vi "Update Metadata using listbox names.vi"(6 "loadStatus Refnum":refnum<vi>, 8 "error in":errorcluster, 10 "Site":string, 11 "RefNumArrIn":refnum<vi>[](array[refnum])) -> (0 "error out":errorcluster, 3 "RefNumArrOut":refnum<vi>[](array[refnum]))   [LabVIEW 2015]
uses:
  <vilib>/addons/database/Connection.llb/DB Tools Open Connec (Path).vi
  <vilib>/addons/database/Connection.llb/Conn Execute.vi
  <vilib>/addons/database/Recordset.llb/Rec Destroy - Connection.vi
  <vilib>/addons/database/NI_Database_API.lvlib
panel:
  out "App.Dir":path
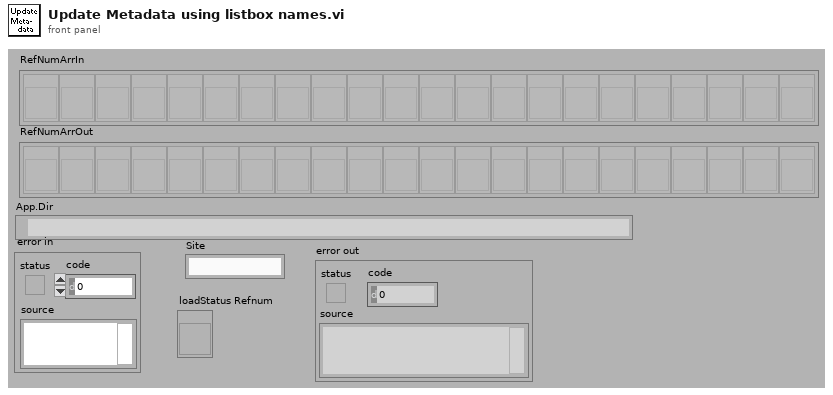
[diagram p1: front panel]
types:
  T1 = typedef "NI_Database_API.lvlib/Conn ObjectReference.ctl" = refnum<k1>
  T2 = typedef "NI_Database_API.lvlib/Rec ObjectReference.ctl" = refnum<k1>
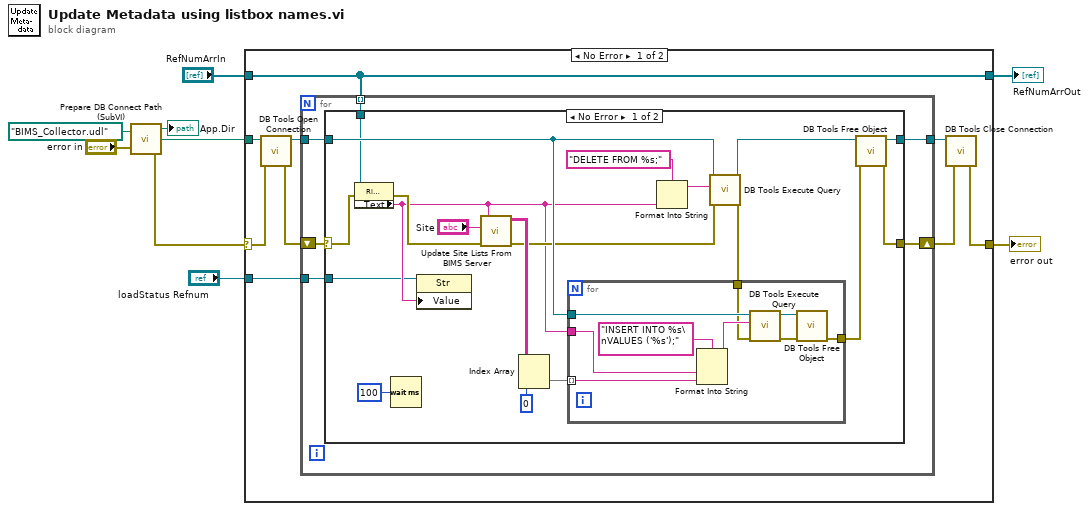
[diagram p0: block diagram]
diagram:
  n1 = call "Prepare DB Connect Path (SubVI).vi"("connectString"=path "BIMS_Collector.udl", "error in"="error in") -> ("App.Dir"=→"App.Dir":path, "appended path"=w9:path, "error out"=w3:errorcluster)
  n2 = case shown="No Error" w3 {
    selector: w3 -> [w13 w55]
    tunnel: w9 -> [w16 _]
    tunnel: [w12 w55] -> w2
    tunnel: "RefNumArrIn" -> [w11 w56]
    tunnel: [w11 w56] -> w6
    tunnel: "loadStatus Refnum" -> [w10 _]
    frame No Error {
      n3 = call-poly <vilib>:"DB Tools Open Connection.vi"("error in (no error)"=w13, "connection information"=w16) -> ("error out"=w18:errorcluster, "connection reference"=w17:T1)  [unwired: 3 in, 3 out]
      n4 = for {
        shift-right: [w23] -> w14
        shift-left: w18 -> [w21]
        tunnel: w17 -> [w22]
        tunnel: [w24] -> w15
        tunnel: w11 -> [w20] mode=indexing
        tunnel: w10 -> [w19]
        n5 = case shown="No Error" w21 {
          selector: w21 -> [w28 w53]
          tunnel: [w43 w54] -> w24
          tunnel: [w42 w53] -> w23
          tunnel: w22 -> [w40 w54]
          tunnel: w20 -> [w30 _]
          tunnel: w19 -> [w26 _]
          frame No Error {
            n6 = property class="Ring (strict)"(reference=w30, error in=w28) -> (error out=w32:errorcluster, "Label.Text"=w27:string)  [unwired: 1 out]
            n7 = Wait (ms)(milliseconds to wait=u32 100) -> ()  [unwired: 1 out]
            n8 = property class="Str"(reference=w26, "Value"=w27) -> ()  [unwired: 1 in, 2 out]
            n9 = call "Update Site Lists From BIMS Server.vi"("error IN"=w32, "Site"="Site", "Lookup Table Name"=w27) -> ("error OUT"=w29:errorcluster, "recordset data"=w31:string[][])  [unwired: 3 out]
            n10 = Index Array(array=w31, index (col)=0 ("disabled index (col)")) -> (element=w41:string[])  [unwired: 1 in]
            n11 = Format Into String(format string="DELETE FROM %s;" ("SQL query"), w27) -> (resulting string=w36:string)  [unwired: 2 in, 1 out]
            n12 = call-poly <vilib>:"DB Tools Execute Query.vi"("error in (no error)"=w29, "SQL query"=w36, "connection reference"=w40) -> ("error out"=w34:errorcluster, "recordset reference"=w39:T2)  [unwired: 1 in, 4 out]
            n13 = for {
              tunnel: w41 -> [w46] mode=indexing
              tunnel: w40 -> [w50]
              tunnel: [w47] -> w38
              tunnel: w34 -> [w45]
              tunnel: w27 -> [w44]
              n14 = Format Into String(format string="INSERT INTO %s\nVALUES ('%s');" ("SQL query"), w44, w46) -> (resulting string=w51:string)  [unwired: 2 in, 1 out]
              n15 = call-poly <vilib>:"DB Tools Execute Query.vi"("error in (no error)"=w45, "SQL query"=w51, "connection reference"=w50) -> ("error out"=w49:errorcluster, "recordset reference"=w48:T2)  [unwired: 1 in, 4 out]
              n16 = call-poly <vilib>:"DB Tools Free Object.vi"("error in (no error)"=w49, "recordset reference"=w48) -> ("error out"=w47:errorcluster)  [unwired: 9 out]
            }
            n17 = call-poly <vilib>:"DB Tools Free Object.vi"("error in (no error)"=w38, "recordset reference"=w39) -> ("error out"=w42:errorcluster, "connection reference"=w43:T1)  [unwired: 8 out]
          }
          frame Error {
          }
        }
      }
      n18 = call <vilib>:"DB Tools Close Connection.vi"("error in (no error)"=w14, "connection reference"=w15) -> ("error out"=w12:errorcluster)  [unwired: 5 out]
    }
    frame Error {
    }
  }
  "error out" <- w2
  "RefNumArrOut" <- w6
